vi "Bus Interface.vi"(0 "AddressSpace":refnum<class "AddressSpace.lvclass">, 1 "abort":bool, 5 "instruction":T2, 9 "input valid":bool) -> (6 "response":T1, 10 "done":bool, 14 "ready for input":bool)   [LabVIEW 2017, in "ScaleAndLimit.lvlib" / "AddressSpace.lvclass"]
uses:
  AddressSpace.lvclass
  <instrlib>/_niInstr/Instruction Framework/v1/FPGA/Interfaces/Address Space/Address Space Instruction.ctl
  <instrlib>/_niInstr/Instruction Framework/v1/FPGA/Typedefs/Response.ctl
  AddressSpace.lvclass/AddressSpace.ctl
  <vilib>/Utility/error.llb/Clear Errors.vi
  <vilib>/rvi/Emulation/niFpgaSctlEmulationGetInTimedLoop.vi
  <vilib>/rvi/Emulation/niFpgaProcessEmulError.vi
  <vilib>/rvi/DataTransferAndStorage/Container/Common/niFpgaContainerGetUniqueNameForEmu.vi
  <vilib>/rvi/Memory/Memory_Emulation/nirvimemoryEmulationManagerCache_SetValue.vi
  <vilib>/rvi/Memory/Memory_Emulation/nirvimemoryEmulationManagerCache_GetValue.vi
  <vilib>/rvi/Memory/Memory_Emulation/nirvimemoryEmulationManagerCache_ReleaseExclusive.vi
  <vilib>/rvi/Memory/Memory_Emulation/nirvimemoryEmulationManagerCache_InsertValue.vi
  <vilib>/rvi/Memory/Memory_Emulation/niFpgaMemoryEmulationValidateCache.vi
  <vilib>/rvi/Memory/Memory_Emulation/nirvimemoryEmulationManagerCache_MakeExclusive.vi
  <vilib>/rvi/Memory/Memory_Emulation/niFpgaMemoryEmulationCacheClearOnFirstRun.vi
  <vilib>/rvi/Emulation/niFpgaEmulationIsFPGAContextNoSignature.vi
  <vilib>/rvi/DataTransferAndStorage/Container/Common/niFpgaContainerExecOnDevCompGetState.vi
  <vilib>/rvi/DataTransferAndStorage/Container/XNode/niFpgaContainer.xnode
  <vilib>/rvi/DataTransferAndStorage/Register/Emulation/niFpgaRegisterEmulationRefIn.vi
  <instrlib>/_niInstr/Instruction Framework/v1/FPGA/Typedefs/niInstr Instruction Framework v1 FPGA.lvlib
  <instrlib>/_niInstr/Instruction Framework/v1/FPGA/Interfaces/Address Space/Address Space.lvclass
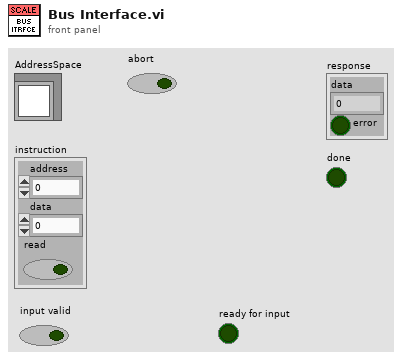
[diagram p1: front panel]
types:
  T1 = typedef "niInstr Instruction Framework v1 FPGA.lvlib/Response.ctl" = cluster{"data":u64, "error":bool}
  T2 = typedef "niInstr Instruction Framework Interfaces v1 FPGA.lvlib/Address Space.lvclass/Address Space Instruction.ctl" = cluster{"address":u32, "data":u64, "read":bool}
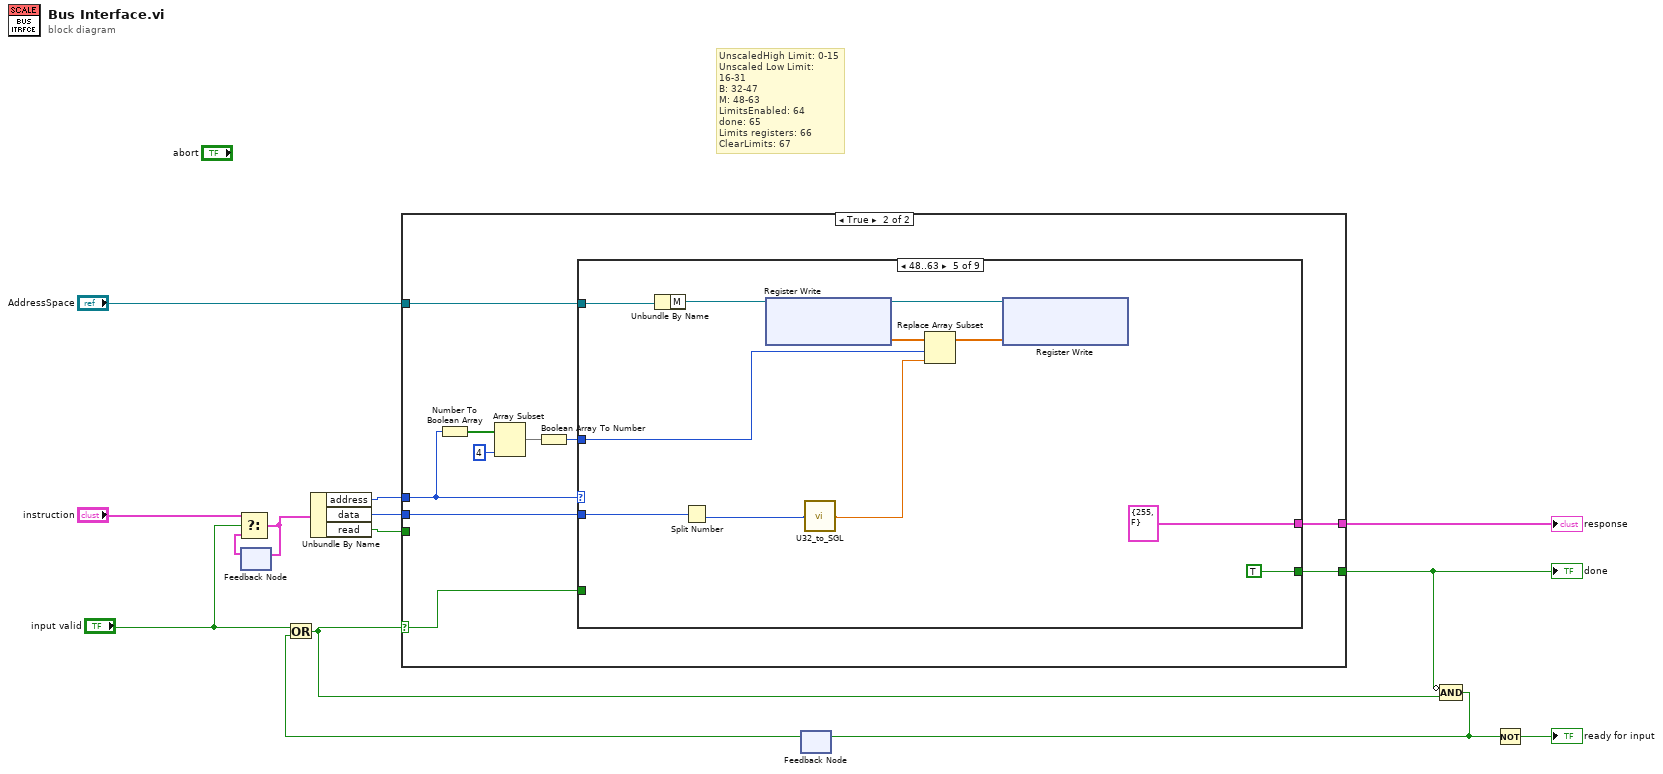
[diagram p0: block diagram]
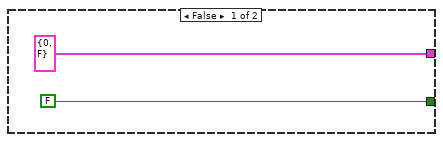
[diagram p2: hidden frame]
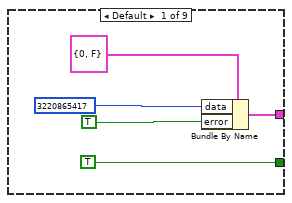
[diagram p3: hidden frame]
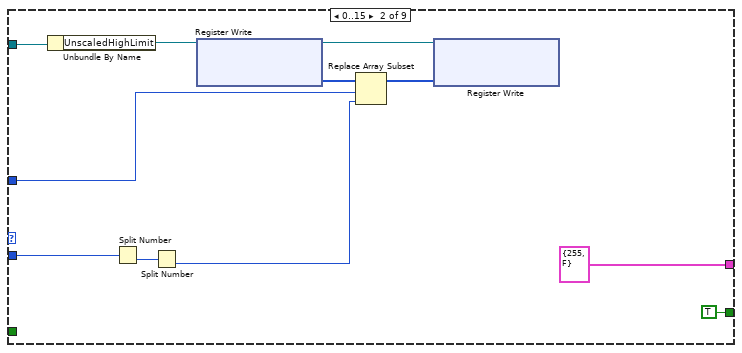
[diagram p4: hidden frame]
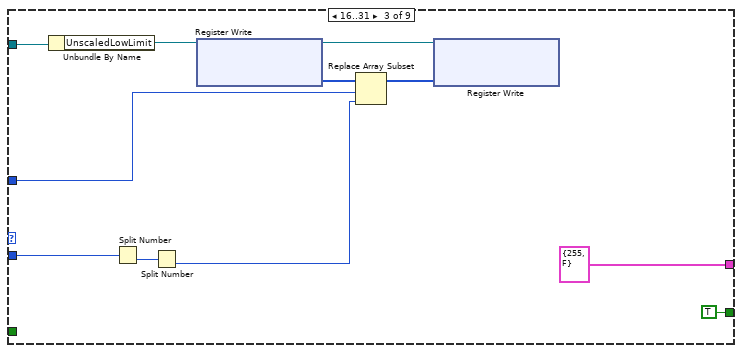
[diagram p5: hidden frame]
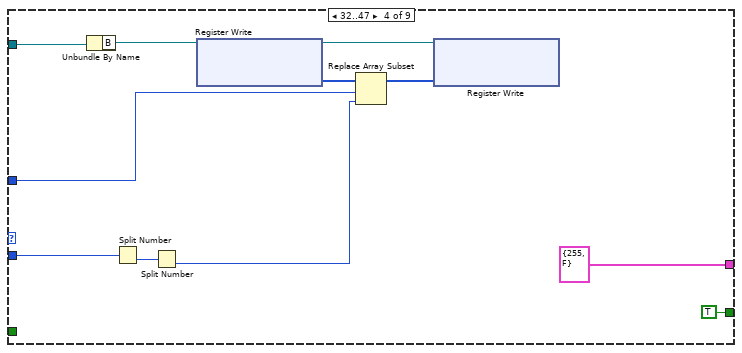
[diagram p6: hidden frame]
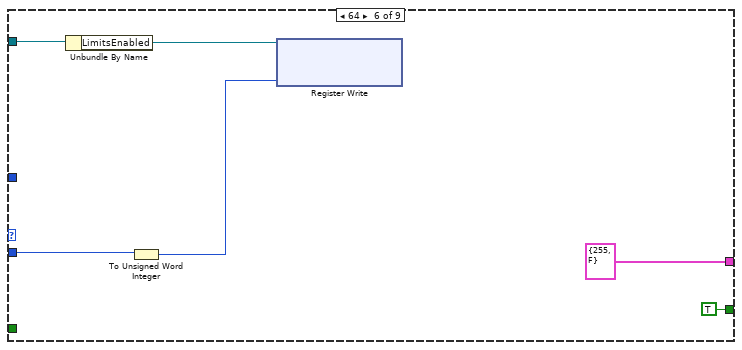
[diagram p7: hidden frame]
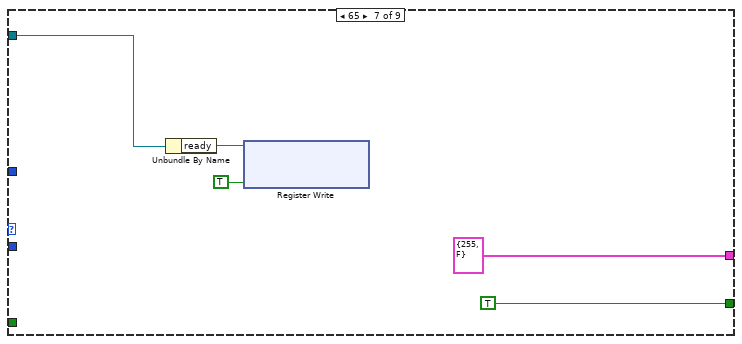
[diagram p8: hidden frame]
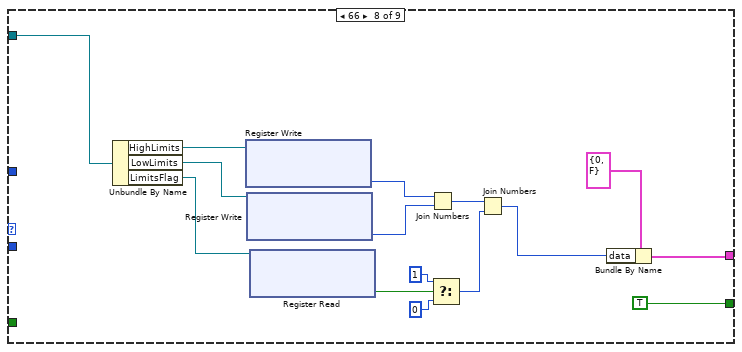
[diagram p9: hidden frame]
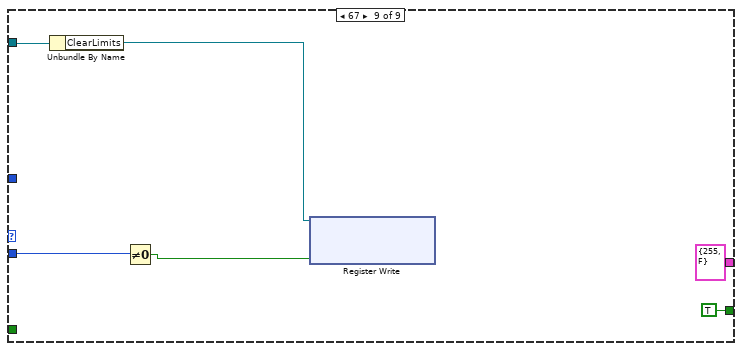
[diagram p10: hidden frame]
diagram:
  # "UnscaledHigh Limit: 0-15\nUnscaled Low Limit: 16-31\nB: 32-47\nM: 48-63\nLimitsEnabled: 64\ndone: 65\nLimits registers: 66\nClearLimits: 67"
  n1 = feedback #1() -> (w14:T2)  [unwired: 1 in]
  n2 = Select(t="instruction", s="input valid", f=w14) -> (s? t:f=w13:T2)
  n3 = feedback-in #1(w13) -> ()
  n4 = Unbundle By Name(w13) -> ("address"=w10:u32, "data"=w11:u64, "read"=w12:bool)
  n5 = feedback #2() -> (w7:bool)  [unwired: 1 in]
  n6 = Or(x="input valid", y=w7) -> (x .or. y?=w8:bool)
  n7 = case shown="True" w8 {
    selector: w8 -> [_ w17]
    tunnel: w12 -> [_ _]
    tunnel: w10 -> [_ w26]
    tunnel: w11 -> [_ w25]
    tunnel: [T1 {"data"=0, "error"=FALSE} ("response") w24] -> w3
    tunnel: [FALSE ("Output Valid") w23] -> w2
    tunnel: "AddressSpace" -> [_ w22]
    frame False {
    }
    frame True {
      n8 = Number To Boolean Array(number=w26) -> (Boolean array=w19:bool[])
      n9 = Array Subset(array=w19, length=4) -> (w21:bool[])  [unwired: 1 in]
      n10 = Boolean Array To Number(Boolean array=w21) -> (number=w18:u8)
      n11 = case shown="48..63" w26 {
        tunnel: w25 -> [_ w39 w50 w61 w72 w78 _ _ w105]
        tunnel: [w28 T1 {"data"=255, "error"=FALSE} ("response") T1 {"data"=255, "error"=FALSE} ("response") T1 {"data"=255, "error"=FALSE} ("response") T1 {"data"=255, "error"=FALSE} ("response") T1 {"data"=255, "error"=FALSE} ("response") T1 {"data"=255, "error"=FALSE} ("response") w93 T1 {"data"=255, "error"=FALSE} ("response")] -> w24
        tunnel: [TRUE ("done") TRUE ("done") TRUE ("done") TRUE ("done") TRUE ("done") TRUE ("done") TRUE ("done") TRUE ("done") TRUE ("done")] -> w23
        tunnel: w22 -> [_ w41 w52 w63 w74 w79 w86 w101 w107]
        tunnel: w17 -> [_ _ _ _ _ _ _ _ _]
        tunnel: w18 -> [_ w32 w43 w54 w68 _ _ _ _]
        frame Default {
          n12 = Bundle By Name(cluster=T1 {"data"=0, "error"=FALSE} ("response"), "data"=u64 3220865417, "error"=TRUE) -> (w28:T1)
        }
        frame 0..15 {
          n13 = Unbundle By Name(w41) -> ("UnscaledHighLimit"=w42:refnum<k21>)
          n14 = Split Number(x=w39) -> (lo(x)=w38:u32)  [unwired: 1 out]
          n15 = Split Number(x=w38) -> (lo(x)=w36:u16)  [unwired: 1 out]
          n16 = xnode ("Register Write")("Register In"=w42) -> ("Data"=w37:i16[], "Register Out"=w40:refnum<k21>)
          n17 = Replace Array Subset(array=w37, new element=w36, index=w32) -> (w35:i16[])
          n18 = xnode ("Register Write")("Data"=w35, "Register In"=w40) -> ()  [unwired: 1 out]
        }
        frame 16..31 {
          n19 = Unbundle By Name(w52) -> ("UnscaledLowLimit"=w53:refnum<k21>)
          n20 = Split Number(x=w50) -> (lo(x)=w49:u32)  [unwired: 1 out]
          n21 = Split Number(x=w49) -> (lo(x)=w47:u16)  [unwired: 1 out]
          n22 = xnode ("Register Write")("Register In"=w53) -> ("Data"=w48:i16[], "Register Out"=w51:refnum<k21>)
          n23 = Replace Array Subset(array=w48, new element=w47, index=w43) -> (w46:i16[])
          n24 = xnode ("Register Write")("Data"=w46, "Register In"=w51) -> ()  [unwired: 1 out]
        }
        frame 32..47 {
          n25 = Unbundle By Name(w63) -> ("B"=w64:refnum<k21>)
          n26 = Split Number(x=w61) -> (lo(x)=w60:u32)  [unwired: 1 out]
          n27 = Split Number(x=w60) -> (lo(x)=w58:u16)  [unwired: 1 out]
          n28 = xnode ("Register Write")("Register In"=w64) -> ("Data"=w59:i16[], "Register Out"=w62:refnum<k21>)
          n29 = Replace Array Subset(array=w59, new element=w58, index=w54) -> (w57:i16[])
          n30 = xnode ("Register Write")("Data"=w57, "Register In"=w62) -> ()  [unwired: 1 out]
        }
        frame 48..63 {
          n31 = Unbundle By Name(w74) -> ("M"=w75:refnum<k21>)
          n32 = Split Number(x=w72) -> (lo(x)=w67:u32)  [unwired: 1 out]
          n33 = xnode ("Register Write")("Register In"=w75) -> ("Data"=w71:sgl[], "Register Out"=w73:refnum<k21>)
          n34 = call <vilib>:"U32_to_SGL.vi"("U32"=w67) -> ("SGL"=w66:sgl)  [unwired: 4 in]
          n35 = Replace Array Subset(array=w71, new element=w66, index=w68) -> (w70:sgl[])
          n36 = xnode ("Register Write")("Data"=w70, "Register In"=w73) -> ()  [unwired: 1 out]
        }
        frame 64 {
          n37 = Unbundle By Name(w79) -> ("LimitsEnabled"=w81:refnum<k21>)
          n38 = To Unsigned Word Integer(number=w78) -> (unsigned 16bit integer=w80:u16)
          n39 = xnode ("Register Write")("Data"=w80, "Register In"=w81) -> ()  [unwired: 1 out]
        }
        frame 65 {
          n40 = Unbundle By Name(w86) -> ("ready"=w85:refnum<k21>)
          n41 = xnode ("Register Write")("Data"=TRUE, "Register In"=w85) -> ()  [unwired: 1 out]
        }
        frame 66 {
          n42 = Unbundle By Name(w101) -> ("HighLimits"=w100:refnum<k21>, "LowLimits"=w98:refnum<k21>, "LimitsFlag"=w92:refnum<k21>)
          n43 = xnode ("Register Write")("Register In"=w100) -> ("Data"=w97:u16)  [unwired: 1 out]
          n44 = xnode ("Register Write")("Register In"=w98) -> ("Data"=w96:u16)  [unwired: 1 out]
          n45 = xnode ("Register Read")("Register In"=w92) -> ("Data"=w90:bool)  [unwired: 1 out]
          n46 = Join Numbers(hi=w97, lo=w96) -> ((hi.lo)=w91:u32)
          n47 = Select(t=u32 1 ("lo"), s=w90, f=u32 0 ("lo")) -> (s? t:f=w87:u32)
          n48 = Join Numbers(hi=w91, lo=w87) -> ((hi.lo)=w94:u64)
          n49 = Bundle By Name(cluster=T1 {"data"=0, "error"=FALSE} ("response"), "data"=w94) -> (w93:T1)
        }
        frame 67 {
          n50 = Unbundle By Name(w107) -> ("ClearLimits"=w106:refnum<k21>)
          n51 = Not Equal To 0?(x=w105) -> (x != 0?=w104:bool)
          n52 = xnode ("Register Write")("Data"=w104, "Register In"=w106) -> ()  [unwired: 1 out]
        }
      }
    }
  }
  "done" <- w2
  "response" <- w3
  n53 = Compound Arithmetic op=AND(invert w2, w8) -> (w9:bool)
  n54 = feedback-in #2(w9) -> ()
  n55 = Not(x=w9) -> (.not. x?=→"ready for input":bool)
